vi "Kaelus PIM Unflatten Driver Configuration.vi"(9 "PIM Configuration (\"\")":string) -> (1 "Configuration":T1={"host IP (localhost)"="localhost", "host Port"=3388, "Model"="", "Serial Number(s)"="", "Calibration Date"=3388.0, "Dual Port?"=FALSE, "DeviceNames"=[], "Parameters"={"TX1start"=0.0, "TX1stop"=0.0, "TX1pmax"=0.0, "TX2start"=0.0, "TX2stop"=0.0, "TX2pmax"=0.0, "RXstart"=0.0, "RXstop"=0.0}, "Interface"=enum."PIM Web Engine"} {"Calibration Date" format="%.2f"; "Parameters"."TX2pmax" format="%.1f"; "Parameters"."TX1pmax" format="%.1f"; "Parameters"."RXstop" format="%.1f"; "Parameters"."RXstart" format="%.1f"; "Parameters"."TX2stop" format="%.1f"; "Parameters"."TX2start" format="%.1f"; "Parameters"."TX1stop" format="%.1f"; "Parameters"."TX1start" format="%.1f"}, 4 "Version":string)   [LabVIEW 2011]
uses:
  PIM Configuration.ctl
  PIM Interface Language.ctl
  PIM Configuration v1.0 - v5.1.ctl
  PIM Configuration v5.2 - v5.3.ctl
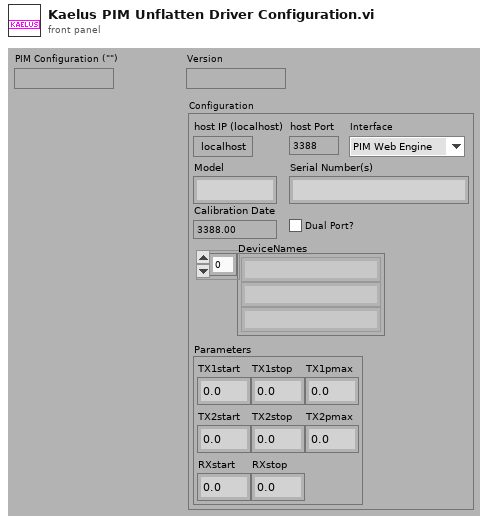
[diagram p1: front panel]
types:
  T1 = typedef "PIM Configuration.ctl" = cluster{"host IP (localhost)":string, "host Port":u16, "Model":string, "Serial Number(s)":string, "Calibration Date":dbl, "Dual Port?":bool, "DeviceNames":string[], "Parameters":cluster{"TX1start":dbl, "TX1stop":dbl, "TX1pmax":dbl, "TX2start":dbl, "TX2stop":dbl, "TX2pmax":dbl, "RXstart":dbl, "RXstop":dbl}, "Interface":T2}
  T2 = typedef "PIM Interface Language.ctl" = enum16{"PIM Web Engine", "PIM HW Engine"}
  T3 = typedef "PIM Configuration v5.2 - v5.3.ctl" = cluster{"host IP (localhost)":string, "host Port":u16, "Model":string, "Serial Number(s)":string, "Calibration Date":dbl, "Dual Port?":bool, "DeviceNames":string[], "Parameters":cluster{"TX1start":dbl, "TX1stop":dbl, "TX1pmax":dbl, "TX2start":dbl, "TX2stop":dbl, "TX2pmax":dbl, "RXstart":dbl, "RXstop":dbl}}
  T4 = typedef "PIM Configuration v1.0 - v5.1.ctl" = cluster{"host IP (localhost)":string, "host Port":u16}
  T5 = cluster{"TX1start":dbl, "TX1stop":dbl, "TX1pmax":dbl, "TX2start":dbl, "TX2stop":dbl, "TX2pmax":dbl, "RXstart":dbl, "RXstop":dbl}
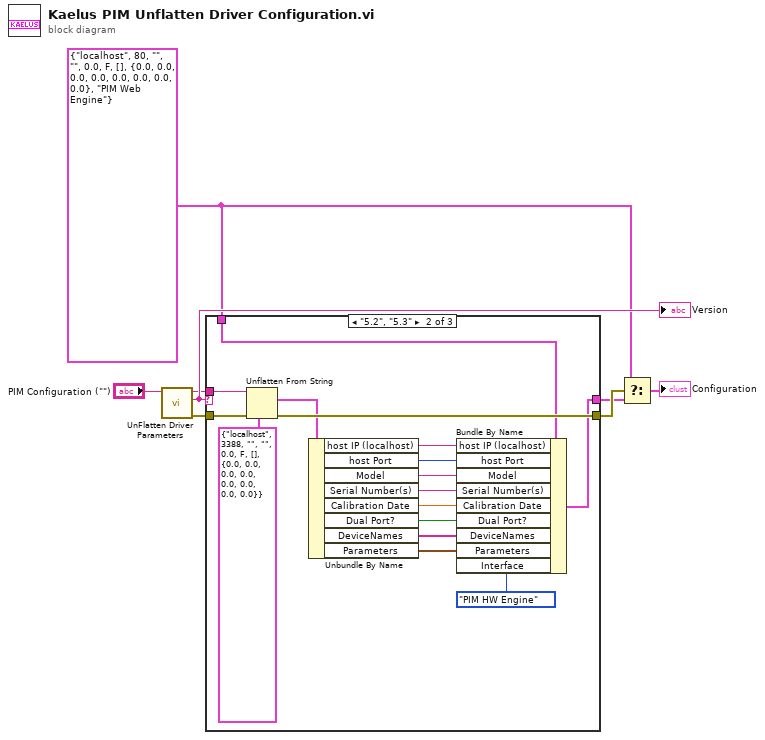
[diagram p0: block diagram]
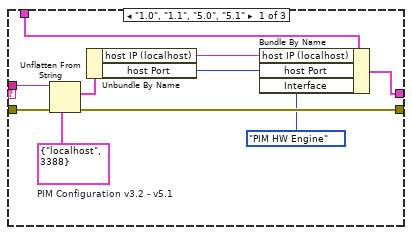
[diagram p2: hidden frame]
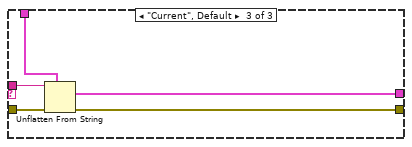
[diagram p3: hidden frame]
diagram:
  w3 = T1 {"host IP (localhost)"="localhost", "host Port"=80, "Model"="", "Serial Number(s)"="", "Calibration Date"=0.0, "Dual Port?"=FALSE, "DeviceNames"=[], "Parameters"={"TX1start"=0.0, "TX1stop"=0.0, "TX1pmax"=0.0, "TX2start"=0.0, "TX2stop"=0.0, "TX2pmax"=0.0, "RXstart"=0.0, "RXstop"=0.0}, "Interface"=enum."PIM Web Engine"} ("PIM Configuration")
  n1 = call "UnFlatten Driver Parameters.vi"("Flattened Driver Parameters with Version (\"\")"="PIM Configuration (\"\")") -> ("error out"=w2:errorcluster, "Driver Version"=w8:string, "Flat Driver Parameters"=w7:string)  [unwired: 1 in, 3 out]
  "Version" <- w8
  n2 = case shown="\"5.2\", \"5.3\"" w8 {
    tunnel: w7 -> [w18 w34 w39]
    tunnel: w3 -> [w14 w31 w38]
    tunnel: [w13 w30 w37] -> w5
    tunnel: [w15 w32 w36] -> w6
    tunnel: w2 -> [w17 w33 w35]
    frame "1.0", "1.1", "5.0", "5.1" {
      w16 = T4 {"host IP (localhost)"="localhost", "host Port"=3388}  # PIM Configuration v3.2 - v5.1
      n3 = Unflatten From String(type=w16, binary string=w18, error in (no error)=w17) -> (value=w12:T4, error out=w15:errorcluster)  [unwired: 3 out]
      n4 = Unbundle By Name(w12) -> ("host IP (localhost)"=w11:string, "host Port"=w10:u16)
      n5 = Bundle By Name(cluster=w14, "host IP (localhost)"=w11, "host Port"=w10, "Interface"=PIM_Interface_Language."PIM HW Engine") -> (w13:T1)
    }
    frame "5.2", "5.3" {
      n6 = Unflatten From String(type=T3 {"host IP (localhost)"="localhost", "host Port"=3388, "Model"="", "Serial Number(s)"="", "Calibration Date"=0.0, "Dual Port?"=FALSE, "DeviceNames"=[], "Parameters"={"TX1start"=0.0, "TX1stop"=0.0, "TX1pmax"=0.0, "TX2start"=0.0, "TX2stop"=0.0, "TX2pmax"=0.0, "RXstart"=0.0, "RXstop"=0.0}} ("PIM Configuration v5.1 - v5.3"), binary string=w34, error in (no error)=w33) -> (value=w27:T3, error out=w32:errorcluster)  [unwired: 3 out]
      n7 = Unbundle By Name(w27) -> ("host IP (localhost)"=w26:string, "host Port"=w25:u16, "Model"=w24:string, "Serial Number(s)"=w23:string, "Calibration Date"=w22:dbl, "Dual Port?"=w21:bool, "DeviceNames"=w20:string[], "Parameters"=w19:T5)
      n8 = Bundle By Name(cluster=w31, "host IP (localhost)"=w26, "host Port"=w25, "Model"=w24, "Serial Number(s)"=w23, "Calibration Date"=w22, "Dual Port?"=w21, "DeviceNames"=w20, "Parameters"=w19, "Interface"=PIM_Interface_Language."PIM HW Engine") -> (w30:T1)
    }
    frame "Current", Default {
      n9 = Unflatten From String(type=w38, binary string=w39, error in (no error)=w35) -> (value=w37:T1, error out=w36:errorcluster)  [unwired: 3 out]
    }
  }
  n10 = Select(t=w3, s=w6, f=w5) -> (s? t:f=→"Configuration":T1)
